vi "GFITS_FillHdrGbl.vi"(6 "mext":bool, 7 "ReadMode":string, 9 "number of Extensions":u16, 10 "def_timing":string="after", 11 "hdrfile":path) -> ()   [LabVIEW 2016]
uses:
  GFITS_Gbls.vi
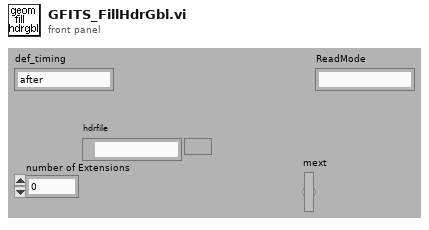
[diagram p1: front panel]
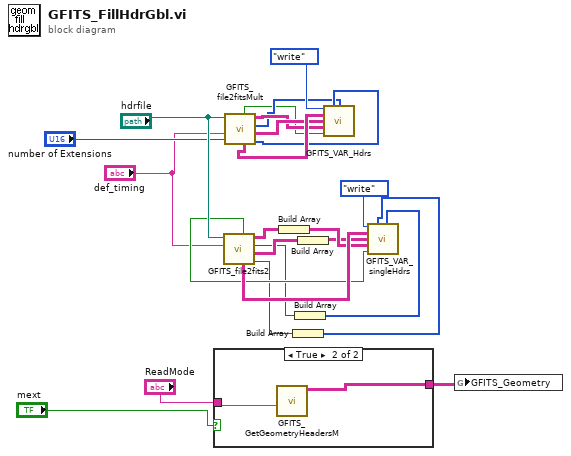
[diagram p0: block diagram]
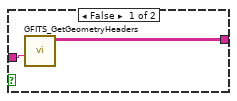
[diagram p2: hidden frame]
diagram:
  n1 = case shown="True" "mext" {
    tunnel: "ReadMode" -> [w26 w28]
    tunnel: [w25 w27] -> w2
    frame False {
      n2 = call "GFITS_GetGeometryHeaders.vi"("readmode"=w26) -> ("Keywords out"=w25:string[][][])  [unwired: 10 out]
    }
    frame True {
      n3 = call "GFITS_GetGeometryHeadersM.vi"("readmode"=w28) -> ("Keywords out"=w27:string[][][])  [unwired: 10 out]
    }
  }
  n4 = call "GFITS_file2fits2.vi"("def_timing"="def_timing", "file"="hdrfile") -> ("number of before keywords"=w8:i32, "before Keywords"=w11:string[][], "number of after keywords"=w7:i32, "after Keywords"=w13:string[][], "all keys"=w14:string[][], "geominfo?"=w9:bool)  [unwired: 4 out]
  n5 = call "GFITS_file2fitsMult.vi"("def_timing"="def_timing", "number of Extensions"="number of Extensions", "filename"="hdrfile") -> ("number of before keys"=w17:i32[], "before keys"=w19:string[][][], "number of keywords"=w16:i32[], "Keywords"=w18:string[][][], "all keys"=w20:string[][][], "geominfo?"=w15:bool)  [unwired: 1 in, 2 out]
  n6 = Build Array(w13) -> (w12:string[][][])
  n7 = Build Array(w8) -> (w5:i32[])
  n8 = Build Array(w7) -> (w6:i32[])
  n9 = Build Array(w11) -> (w10:string[][][])
  n10 = call "GFITS_VAR_Hdrs.vi"("action"=enum16{"read", "write"}."write", "nkeys before in"=w17, "nkeys after in"=w16, "GFITS_allkeys in"=w20, "GFITS_beforein"=w19, "GFITS_after in"=w18, "geom info in"=w15) -> ()  [unwired: 9 out]
  n11 = call "GFITS_VAR_singleHdrs.vi"("action"=enum16{"read", "write"}."write", "nkeys before in"=w5, "nkeys after in"=w6, "GFITS_allkeys in"=w14, "GFITS_beforein"=w10, "GFITS_after in"=w12, "geom info in"=w9) -> ()  [unwired: 9 out]
  n12 = global write "GFITS_Gbls.vi" "GFITS_Geometry"(w2) -> ()
